vi "USRP Packet Receiver.vi"() -> ()   [LabVIEW 2015]
uses:
  <instrlib>/niUSRP/niUSRP Fetch Rx Data (CDB Cluster).vi
  <vilib>/addons/Modulation/niDMT.lvlib
panel:
  out "Symbol Rate\n[symbols/sec]":dbl=25000.0 format="%#.6p"
  in  "synchronization parameters":T1={"expected sync location (symbols)"=-1, "sync sequence"=[], "sync location uncertainty (symbols)"=0, "sync indent (symbols)"=0} {"sync sequence" format="%.2f"}
  in  "stop":bool
  in  "Tab Control":T2(tab)=enum."Rx Display"
  in  "Acquisition Duration [sec]":dbl=0.04 format="%#.6p"
  in  "Rx Parameters":T3={"Rx IQ Sampling\nRate [s/sec]"=400000.0, "Rx\nFrequency [Hz]"=915000000.0, "Rx Gain [dB]"=20.0, "Rx Antenna"="RX1"} {"Rx Gain [dB]" format="%#.6p"; "Rx\nFrequency [Hz]" format="%#.6p"; "Rx IQ Sampling\nRate [s/sec]" format="%#.6p"}
  out "Actual Rx Parameters":T3={"Rx IQ Sampling\nRate [s/sec]"=200000.0, "Rx\nFrequency [Hz]"=915000000.0, "Rx Gain [dB]"=20.0, "Rx Antenna"="RX1"} {"Rx Gain [dB]" format="%#.6p"; "Rx\nFrequency [Hz]" format="%#.6p"; "Rx IQ Sampling\nRate [s/sec]" format="%#.6p"}
  in  "USRP IP Address":refnum<k15>="192.168.10.3"
  in  "Choose a PSK Format":T4(tab)=enum."QPSK" caption="PSK"
  in  "BPSK System Parameters":T5={"Samples per Symbol"=8, "symbol map"=[], "Differential PSK"=enum."disable", "PSK type"=0} {"PSK type" items=["normal", "shifted", "offset"]; "symbol map" format="%.3f"}
  in  "QPSK System Parameters":T5={"Samples per Symbol"=8, "symbol map"=[], "Differential PSK"=enum."disable", "PSK type"=0} {"PSK type" items=["normal", "shifted", "offset"]; "symbol map" format="%.3f"}
  in  "pi/4 DQPSK System Parameters":T5={"Samples per Symbol"=8, "symbol map"=[], "Differential PSK"=enum."enable", "PSK type"=1} {"PSK type" items=["normal", "shifted", "offset"]; "symbol map" format="%.3f"}
  in  "OQPSK System Parameters":T5={"Samples per Symbol"=8, "symbol map"=[], "Differential PSK"=enum."disable", "PSK type"=2} {"PSK type" items=["normal", "shifted", "offset"]; "symbol map" format="%.3f"}
  in  "8-PSK System Parameters":T5={"Samples per Symbol"=8, "symbol map"=[], "Differential PSK"=enum."disable", "PSK type"=0} {"PSK type" items=["normal", "shifted", "offset"]; "symbol map" format="%.3f"}
  in  "16-PSK System Parameters":T5={"Samples per Symbol"=8, "symbol map"=[], "Differential PSK"=enum."disable", "PSK type"=0} {"PSK type" items=["normal", "shifted", "offset"]; "symbol map" format="%.3f"}
  in  "M":i32=4 min=2 step=2
  in  "Custom System Parameters":T5={"Samples per Symbol"=8, "symbol map"=[], "Differential PSK"=enum."disable", "PSK type"=0} {"PSK type" items=["normal", "shifted", "offset"]; "symbol map" format="%.3f"}
  in  "filter parameters":T6={"Alpha"=0.5, "Filter Length"=6, "TX Filter"=enum."Root Raised Cos"} caption="Matching Filter Parameters" {"Alpha" format="%.2f"}
  in  "PN Sequence Order\nfor Sync":i32=31
  in  "Packet Parameters":T7={"Guard Bits "=30, "Sync Bits"=20, "Message Bits"=128, "Number of Packets \nto Expect"=46}
  out "Recovered Message":string
  out "Received Signal (Raw)":dbl[](graph)
  out "Constellation Graph":T8(graph)
  out "Sync Found":bool
  out "Correct Packets Rx":i16
  in  "Continuous Acquire?":bool
  out "Singal & Noise Power":cluster{"signal_power":dbl, "noise_power":dbl}={"signal_power"=1.4546950663593878e-09, "noise_power"=2.571229598792933e-12}
  out "error out":errorcluster={"status"=FALSE, "code"=1074118647, "source"="niUSRP Fetch Rx Data (CDB Cluster).vi<ERR>Overflow: an internal receive buffer has filled before the data could be returned.  Consider reducing the IQ rate, increasing the Fetch rate, or increasing the number of samples per Fetch."}
  out "Cumulative Packets Recovered":i16(graph)
  out "Signal and Noise Power Tracking":cluster{"total_power":dbl, "noise_power":dbl}(graph)={"total_power"=1.4546950663593878e-09, "noise_power"=2.571229598792933e-12}
  # "Packet Receiver"
  # "Guard\nBand"
  # "Sync\nSeq"
  # "Packet\nNumber"
  # "Pad\nData"
  # "Blank\nFrame"
  # "Data"
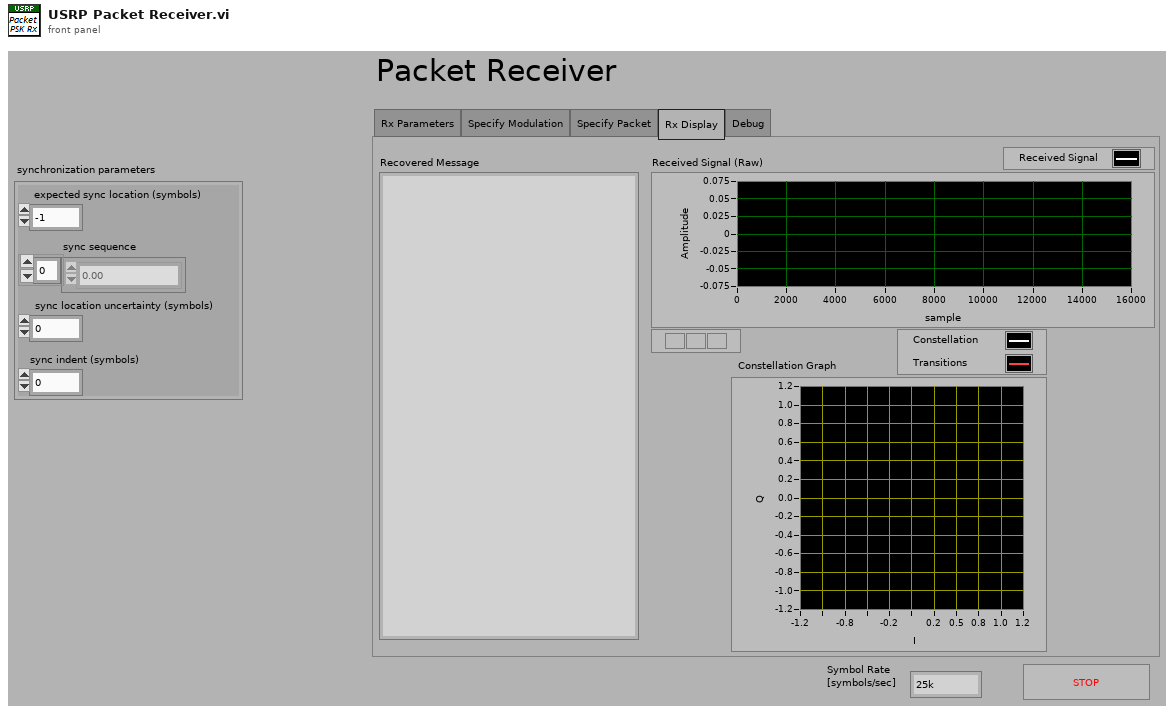
[diagram p1: front panel]
types:
  T1 = cluster{"expected sync location (symbols)":i32, "sync sequence":cdb[], "sync location uncertainty (symbols)":i32, "sync indent (symbols)":i32}
  T2 = enum32{"Rx Parameters", "Specify Modulation", "Specify Packet", "Rx Display", "Debug"}
  T3 = cluster{"Rx IQ Sampling\nRate [s/sec]":dbl, "Rx\nFrequency [Hz]":dbl, "Rx Gain [dB]":dbl, "Rx Antenna":string}
  T4 = enum32{"BPSK", "QPSK", "pi/4DQPSK", "OQPSK", "8-PSK", "16-PSK", "Custom"}
  T5 = cluster{"Samples per Symbol":i32, "symbol map":cdb[], "Differential PSK":enum16{"disable", "enable"}, "PSK type":u16}
  T6 = cluster{"Alpha":dbl, "Filter Length":i32, "TX Filter":enum16{"none", "Raised Cosine", "Root Raised Cos", "Gaussian"}}
  T7 = cluster{"Guard Bits ":i32, "Sync Bits":i32, "Message Bits":i32, "Number of Packets \nto Expect":i32}
  T8 = cluster{"Decimated Array":dbl[], "Decimated Array":dbl[]}[]
  T9 = cluster{"Packet Array":i32[][], "IP Array of Pkt Nums Received  ":bool[]}
  T10 = cluster{"bit stream ":i8[][], "Sync Valid?":bool[], "Decoded Pkt Numbers":u32[], "Enable?":bool}
  T11 = cluster{"packet_arr":cdb[][], "Packets Valid?":bool}
  T12 = cluster{"PSK type":u16, "Samples per Symbol":i32, "Differential PSK":enum16{"disable", "enable"}, "M":i32}
  T13 = cluster{"PSK system parameters":cluster{"samples per symbol (16)":i32, "symbol map":cdb[], "differential PSK":enum16{"disable", "enable"}, "PSK type":u16}, "pulse shaping filter coefficients":dbl[], "matched filter coefficients":dbl[], "synchronization parameters":cluster{"expected sync location (symbols)":i32, "sync sequence":cdb[], "sync location uncertainty (symbols)":i32, "sync indent (symbols)":i32}, "Sync Bits":i8[]}
  T14 = typedef "niAMT.lvlib/Complex Data Waveform.ctl" = cluster{"t0":dbl, "dt":dbl, "Y":cdb[]}
  T15 = cluster{"constellation":dbl[], "oversampled data":dbl[]}[]
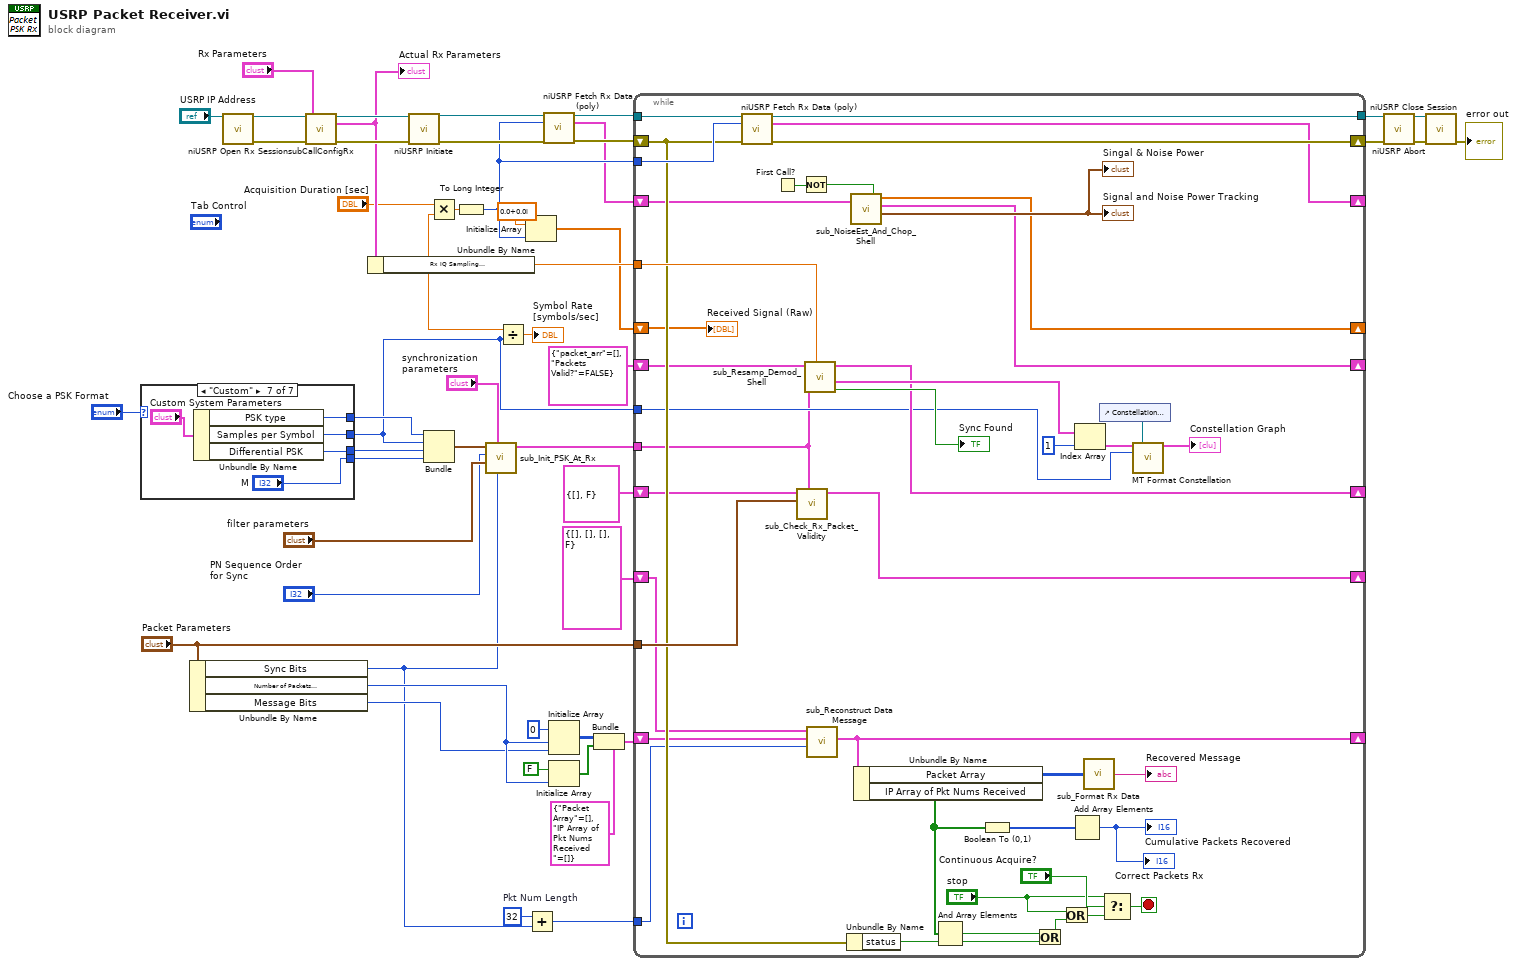
[diagram p0: block diagram]
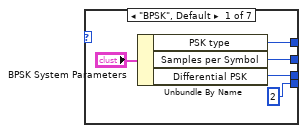
[diagram p2: hidden frame]
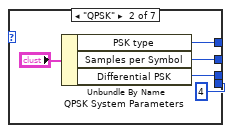
[diagram p3: hidden frame]
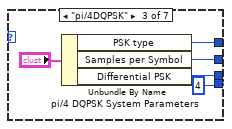
[diagram p4: hidden frame]
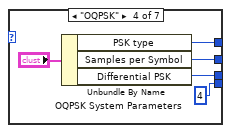
[diagram p5: hidden frame]
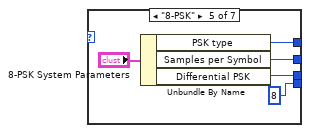
[diagram p6: hidden frame]
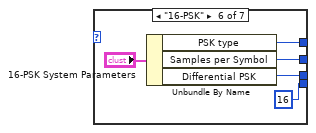
[diagram p7: hidden frame]
diagram:
  w25 = 32  # Pkt Num Length
  n1 = case shown="\"Custom\"" "Choose a PSK Format" {
    tunnel: [w52 w58 w63 w68 w73 w79 w82] -> w22
    tunnel: [w53 w56 w62 w67 w72 w78 w83] -> w33
    tunnel: [2 ("M-PSK (4)") 4 ("M-PSK (4)") 4 ("M-PSK (4)") 4 ("M-PSK (4)") 8 ("M-PSK (4)") 16 ("M-PSK (4)") "M"] -> w32
    tunnel: [w54 w57 w61 w66 w74 w77 w84] -> w34
    frame "BPSK", Default {
      n2 = Unbundle By Name("BPSK System Parameters") -> ("PSK type"=w54:u16, "Samples per Symbol"=w52:i32, "Differential PSK"=w53:enum16{"disable", "enable"})
    }
    frame "QPSK" {
      n3 = Unbundle By Name("QPSK System Parameters") -> ("PSK type"=w57:u16, "Samples per Symbol"=w58:i32, "Differential PSK"=w56:enum16{"disable", "enable"})
    }
    frame "pi/4DQPSK" {
      n4 = Unbundle By Name("pi/4 DQPSK System Parameters") -> ("PSK type"=w61:u16, "Samples per Symbol"=w63:i32, "Differential PSK"=w62:enum16{"disable", "enable"})
    }
    frame "OQPSK" {
      n5 = Unbundle By Name("OQPSK System Parameters") -> ("PSK type"=w66:u16, "Samples per Symbol"=w68:i32, "Differential PSK"=w67:enum16{"disable", "enable"})
    }
    frame "8-PSK" {
      n6 = Unbundle By Name("8-PSK System Parameters") -> ("PSK type"=w74:u16, "Samples per Symbol"=w73:i32, "Differential PSK"=w72:enum16{"disable", "enable"})
    }
    frame "16-PSK" {
      n7 = Unbundle By Name("16-PSK System Parameters") -> ("PSK type"=w77:u16, "Samples per Symbol"=w79:i32, "Differential PSK"=w78:enum16{"disable", "enable"})
    }
    frame "Custom" {
      n8 = Unbundle By Name("Custom System Parameters") -> ("PSK type"=w84:u16, "Samples per Symbol"=w82:i32, "Differential PSK"=w83:enum16{"disable", "enable"})
    }
  }
  n9 = Unbundle By Name("Packet Parameters") -> ("Sync Bits"=w10:i32, "Number of Packets \nto Expect"=w24:i32, "Message Bits"=w23:i32)
  n10 = call <instrlib>:"niUSRP Open Rx Session.vi"("device names"="USRP IP Address") -> ("session handle out"=w45:refnum<k15>, "error out"=w46:errorcluster)  [unwired: 13 in]
  n11 = call "subCallConfigRx.vi"("session handle"=w45, "Rx Parameters"="Rx Parameters", "error in"=w46) -> ("session handle out"=w43:refnum<k15>, "Actual Rx Parameters"=w26:T3, "error out"=w42:errorcluster)  [unwired: 10 in]
  "Actual Rx Parameters" <- w26
  n12 = Unbundle By Name(w26) -> ("Rx IQ Sampling\nRate [s/sec]"=w19:dbl)
  n13 = call <instrlib>:"niUSRP Initiate.vi"("session handle"=w43, "error in (no error)"=w42) -> ("session handle out"=w6:refnum<k15>, "error out"=w5:errorcluster)  [unwired: 12 in]
  n14 = Bundle("PSK type"=w34, "Samples per Symbol"=w22, "Differential PSK"=w33, "M"=w32) -> (w30:T12)  [unwired: 1 in]
  n15 = Multiply(x="Acquisition Duration [sec]", y=w19) -> (x*y=w48:dbl)
  n16 = To Long Integer(number=w48) -> (32bit integer=w4:i32)
  n17 = call "sub_Init_PSK_At_Rx.vi"("Sync Bits"=w10, "synchronization parameters"="synchronization parameters", "filter parameters"="filter parameters", "PN sequence order (9)"="PN Sequence Order\nfor Sync", "PSK Parameters"=w30) -> ("PSK Init Parameters"=w29:T13)  [unwired: 5 in, 1 out]
  n18 = Divide(x=w19, y=w22) -> (x/y=→"Symbol Rate\n[symbols/sec]":dbl)
  n19 = Initialize Array(cdb 0.0+0.0i ("element"), w4) -> (w12:cdb[])
  n20 = Add(x=w25, y=w10) -> (x+y=w35:i32)
  n21 = call-poly <instrlib>:"niUSRP Fetch Rx Data (poly).vi"("session handle"=w6, "number of samples"=w4, "error in (no error)"=w5) -> ("session handle out"=w8:refnum<k15>, "data"=w3:cluster{"t0":dbl, "dt":dbl, "Y":cdb[]}, "error out"=w7:errorcluster)  [unwired: 9 in, 1 out]
  n22 = Initialize Array(0, w24, w23) -> (w14:i32[][])
  n23 = Initialize Array(FALSE, w24) -> (w13:bool[])
  n24 = Bundle(cluster=T9 {"Packet Array"=[], "IP Array of Pkt Nums Received  "=[]} ("Packet Info"), "Packet Array"=w14, "IP Array of Pkt Nums Received"=w13) -> (w1:T9)
  n25 = while {
    tunnel: w19 -> [w127]
    tunnel: w8 -> [w109]
    tunnel: [w107] -> w39
    tunnel: w4 -> [w106]
    tunnel: "Packet Parameters" -> [w126]
    tunnel: w35 -> [w93]
    tunnel: w29 -> [w86]
    shift-right: [w108] -> w38
    shift-left: w7 -> [w104]
    tunnel: w22 -> [w87]
    shift-right: [w91] -> _
    shift-left: w1 -> [w94]
    shift-right: [w100] -> _
    shift-left: T11 {"packet_arr"=[], "Packets Valid?"=FALSE} -> [w101]
    shift-right: [w96] -> _
    shift-left: cluster{"bit stream":i8[][], "Enable?":bool} {"bit stream"=[], "Enable?"=FALSE} ("Output Bitstream") -> [w99]
    shift-right: [w85] -> _
    shift-left: T10 {"bit stream "=[], "Sync Valid?"=[], "Decoded Pkt Numbers"=[], "Enable?"=FALSE} ("Output Bit Stream") -> [w95]
    shift-right: [w97] -> _
    shift-left: w3 -> [w98]
    shift-right: [w88] -> _
    shift-left: w12 -> [w89]
    stop <- w122 stop-if-true
    n26 = call-poly <instrlib>:"niUSRP Fetch Rx Data (poly).vi"("session handle"=w109, "number of samples"=w106, "error in (no error)"=w104) -> ("session handle out"=w107:refnum<k15>, "data"=w97:cluster{"t0":dbl, "dt":dbl, "Y":cdb[]}, "error out"=w108:errorcluster)  [unwired: 9 in, 1 out]
    n27 = First Call?() -> (First Call?: T/F=w112:bool)
    n28 = call "sub_Check_Rx_Packet_Validity.vi"("PSK Init Parameters"=w86, "Packet Parameters"=w126, "Input Bit Stream"=w99) -> ("Output Bit Stream"=w85:T10)  [unwired: 7 in]
    n29 = Not(x=w112) -> (.not. x?=w111:bool)
    n30 = call "sub_Resamp_Demod_Shell.vi"("Rx IQ Sampling\nRate [s/sec]"=w127, "PSK Init Parameters"=w86, "Input Packets"=w101) -> ("Synch Found?"=→"Sync Found":bool, "recovered complex waveform"=w115:T14[], "Output Bitstream"=w96:cluster{"bit stream":i8[][], "Enable?":bool})  [unwired: 3 in]
    n31 = call "sub_Reconstruct Data Message.vi"("Start Loc of Data"=w93, "Packet Info"=w94, "Input Stream"=w95) -> ("Packet Info out"=w91:T9)  [unwired: 8 in]
    n32 = Unbundle By Name(w104) -> ("status"=w103:bool)
    n33 = call "sub_NoiseEst_And_Chop_Shell.vi"("data"=w98, "Enable"=w111) -> ("Singal & Noise Power"=→"Signal and Noise Power Tracking" →"Singal & Noise Power":cluster{"signal_power":dbl, "noise_power":dbl}, "Output Packets"=w100:cluster{"Packets":cdb[][], "Enable?":bool}, "Delay signal (for plotting use only)"=w88:cdb[])  [unwired: 3 in]
    n34 = Unbundle By Name(w91) -> ("Packet Array"=w92:i32[][], "IP Array of Pkt Nums Received"=w90:bool[])
    n35 = And Array Elements(Boolean array=w90) -> (logical AND=w105:bool)
    n36 = Boolean To (0,1)(Boolean=w90) -> (0, 1=w125:i16[])
    n37 = Or(x=w105, y=w103) -> (x .or. y?=w102:bool)
    n38 = Or(x="stop", y=w102) -> (x .or. y?=w123:bool)
    n39 = Add Array Elements(numeric array=w125) -> (sum=→"Correct Packets Rx" →"Cumulative Packets Recovered":i16)
    n40 = Index Array(array=w115, index=1) -> (element=w114:T14)
    n41 = call "sub_Format Rx Data.vi"("Output Packet Array"=w92) -> ("Received Message"=→"Recovered Message":string)
    n42 = control-ref of="Constellation Graph"() -> (w117:refnum<vi>)
    n43 = Select(t="stop", s="Continuous Acquire?", f=w123) -> (s? t:f=w122:bool)
    n44 = call <vilib>:"MT Format Constellation.vi"("waveform"=w114, "constellation reference"=w117, "samples per symbol"=w87) -> ("constellation graph"=→"Constellation Graph":T15)  [unwired: 2 in, 10 out]
    "Received Signal (Raw)" <- w89
  }
  n45 = call <instrlib>:"niUSRP Abort.vi"("session handle"=w39, "error in (no error)"=w38) -> ("session handle out"=w40:refnum<k15>, "error out"=w41:errorcluster)  [unwired: 12 in]
  n46 = call <instrlib>:"niUSRP Close Session.vi"("session handle"=w40, "error in (no error)"=w41) -> ("error out"=→"error out":errorcluster)  [unwired: 13 in]
